vi "DblToGString.vi"(1 "Numeric":dbl) -> (0 "String":string)   [LabVIEW 2024]
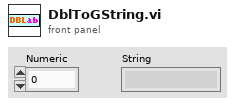
[diagram p1: front panel]
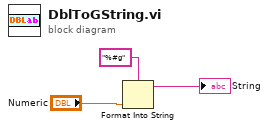
[diagram p0: block diagram]
diagram:
  n1 = Format Into String(format string="%#g", "Numeric") -> (resulting string=→"String":string)  [unwired: 2 in, 1 out]
